vi "initialize.vi"(0 "HGF_DSCSubscriber in":refnum<class "HGF_DSCSubscriber.lvclass">, 3 "initializationData":variant, 5 "error in (no error)":errorcluster, 7 "binaryString":string, 8 "I8 Array":i8[](array[numeric]), 9 "prependSize? (T)":bool, 11 "byteOrder (0:big-endian, network order)":T1(ring)) -> (14 "HGF_DSCSubscriber out":refnum<class "HGF_DSCSubscriber.lvclass">, 17 "found?":bool, 19 "error out":errorcluster)   [LabVIEW 2012, in "HGF_DSC.lvlib" / "HGF_DSCSubscriber.lvclass"]
uses:
  HGF_DSCSubscriber.lvclass
  HGF_SV/HGF_SVSubscriber/HGF_SVSubscriber.lvclass
  HGF_DSCSubscriber.lvclass/HGF_DSCSubscriber.ctl
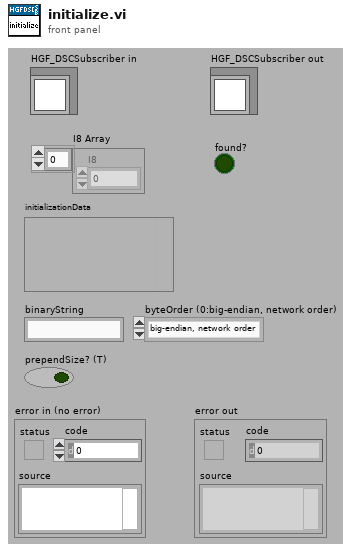
[diagram p1: front panel]
types:
  T1 = enum16{"big-endian, network order", "native, host order", "little-endian"}
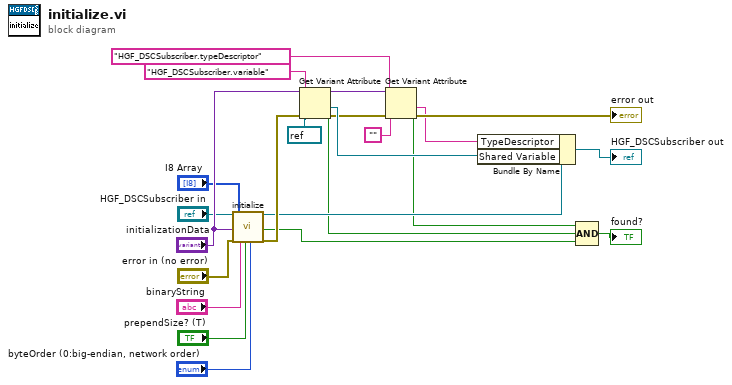
[diagram p0: block diagram]
diagram:
  n1 = call-parent "initialize.vi"("HGF_SVSubscriber in"="HGF_DSCSubscriber in", "initializationData"="initializationData", "error in (no error)"="error in (no error)", "binaryString"="binaryString", "I8 Array"="I8 Array", "prependSize? (T)"="prependSize? (T)", "byteOrder (0:big-endian, network order)"="byteOrder (0:big-endian, network order)") -> ("HGF_SVSubscriber out"=w15:refnum<class "HGF_DSCSubscriber.lvclass">, "found?"=w14:bool, "error out"=w23:errorcluster)  [unwired: 10 out]
  n2 = Get Variant Attribute(Variant="initializationData", name="HGF_DSCSubscriber.variable", default value (empty Variant)=refnum<k21> refnum, error in=w23) -> (duplicate Variant=w3:variant, found=w10:bool, value=w8:refnum<k21>, error out=w7:errorcluster)
  n3 = Get Variant Attribute(Variant=w3, name="HGF_DSCSubscriber.typeDescriptor", default value (empty Variant)="", error in=w7) -> (found=w1:bool, value=w2:string, error out=→"error out":errorcluster)  [unwired: 1 out]
  n4 = Bundle By Name(cluster=w15, "TypeDescriptor"=w2, "Shared Variable"=w8) -> (→"HGF_DSCSubscriber out":refnum<class "HGF_DSCSubscriber.lvclass">)
  n5 = Compound Arithmetic op=AND(w1, w10, w14) -> (→"found?":bool)
